vi "daq_sound_output.vi"() -> ()   [LabVIEW 2022 SP3]
uses:
  typedefs/state_control.ctl
  <vilib>/DAQmx/write.llb/DAQmx Write (Analog Wfm 1Chan NSamp).vi
  <vilib>/DAQmx/create/channels.llb/DAQmx Create Channel (AO-Voltage-Basic).vi
  <vilib>/sound2/lvsound2.llb/Sound File Read Open.vi
  <vilib>/sound2/lvsound2.llb/Sound File Info (refnum).vi
  <vilib>/DAQmx/configure/timing.llb/DAQmx Timing (Sample Clock).vi
  <vilib>/DAQmx/miscellaneous.llb/DAQmx Fill In Error Info.vi
panel:
  in  "Strain Gauge":tag="cDAQ4Mod1/ai0"
  in  "Thermocouple":tag="cDAQ4Mod2/ai0"
  in  "Play\nButton":bool
  in  "Trigger source in":tag="/cDAQ4/PFI0"
  in  "Trigger counter":tag="cDAQ4/_ctr0"
  in  "LEDs":tag="cDAQ4Mod3/port0/line0:7"
  in  "stop":bool
  in  "Path":path=path "C:/Users/Dell NI/Desktop/SoundEditor/data/39;SING, SING, SING39; BY BENNY GOODMAN-YoutubeConvert.cc.wav"
  in  "Audio Output":tag="cDAQ4Mod4/ao0"
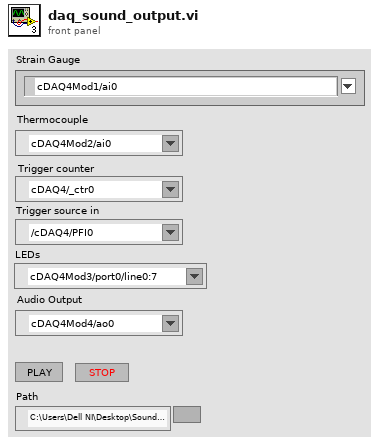
[diagram p1: front panel]
types:
  T1 = typedef "state_control.ctl" = enum16{"Running", "Stopped", "Forwarding"}
  T2 = typedef "Sound File Refnum.ctl" = refnum<file>
  T3 = typedef "Sound Data Format.ctl" = cluster{"sample rate (S/s)":dbl, "number of channels":i32, "bits per sample":i32}
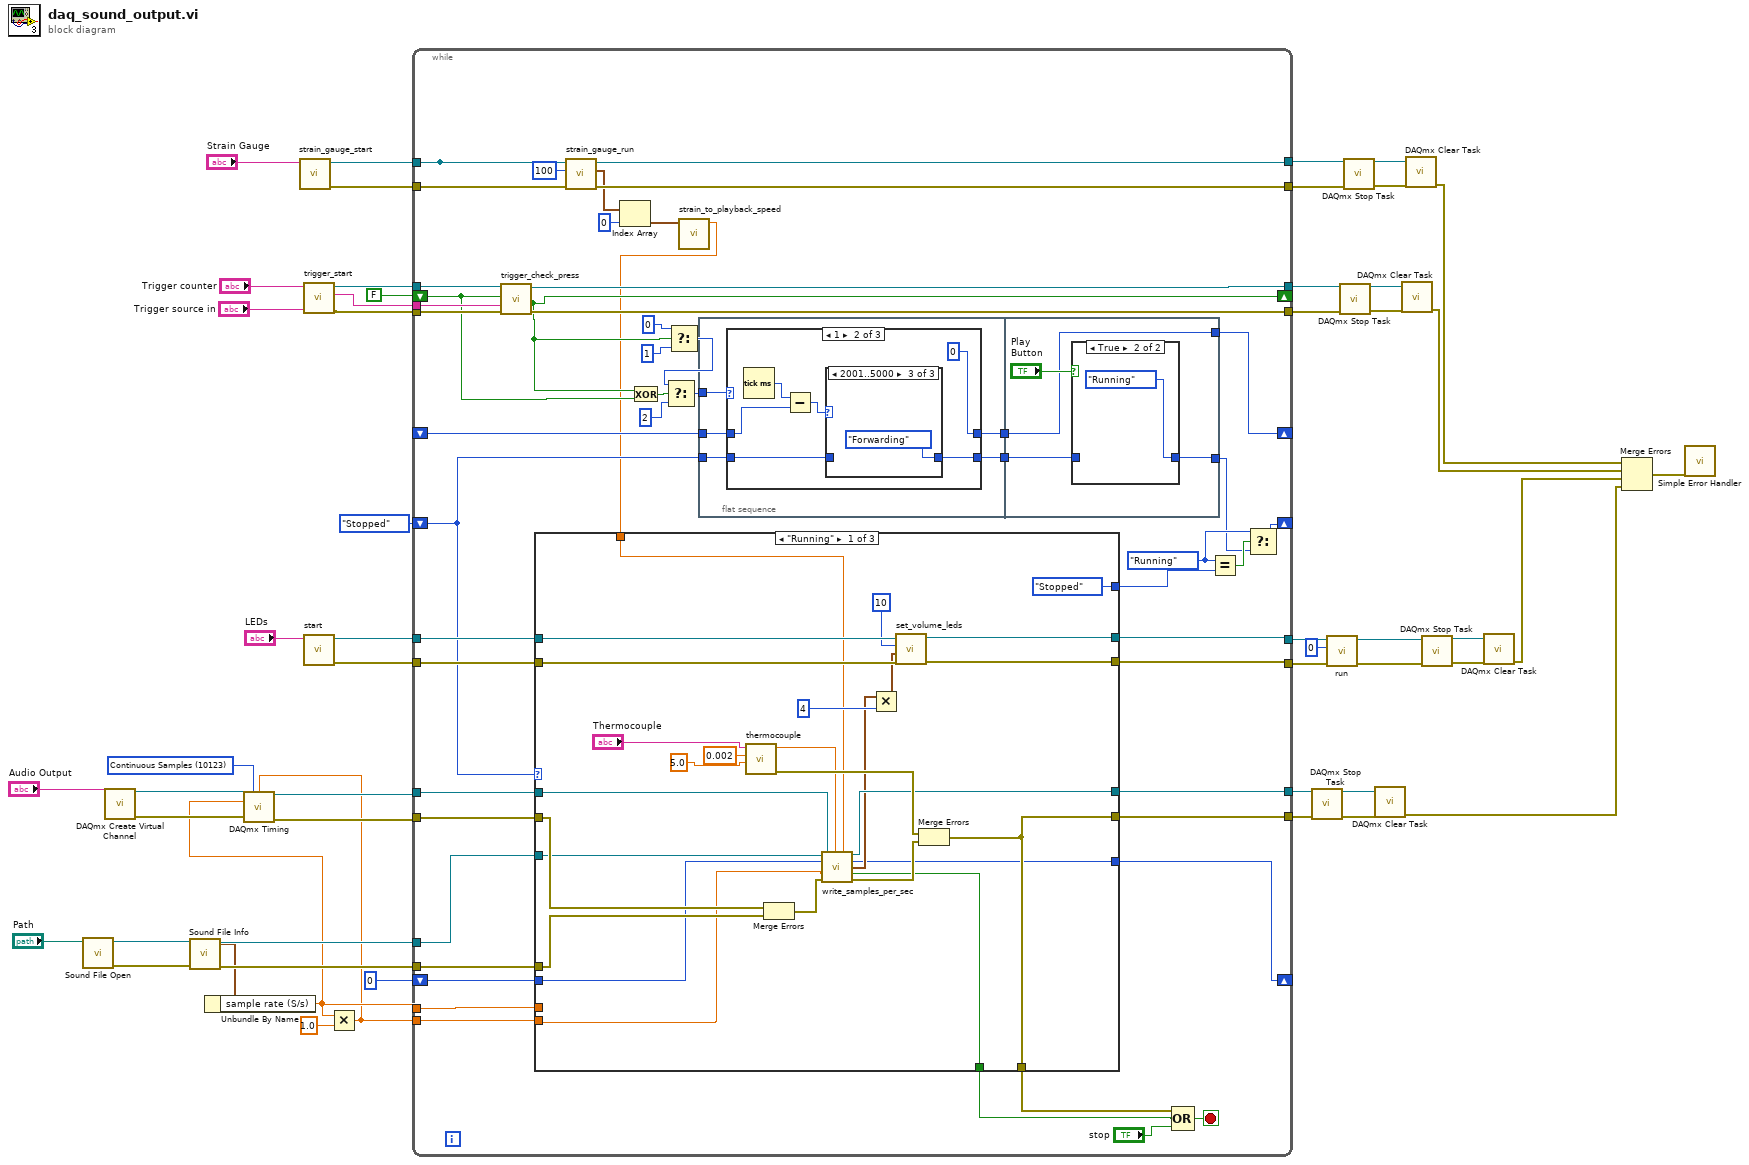
[diagram p0: block diagram]
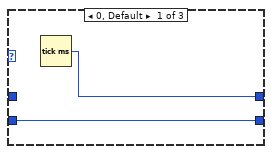
[diagram p2: hidden frame]
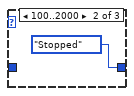
[diagram p4: hidden frame]
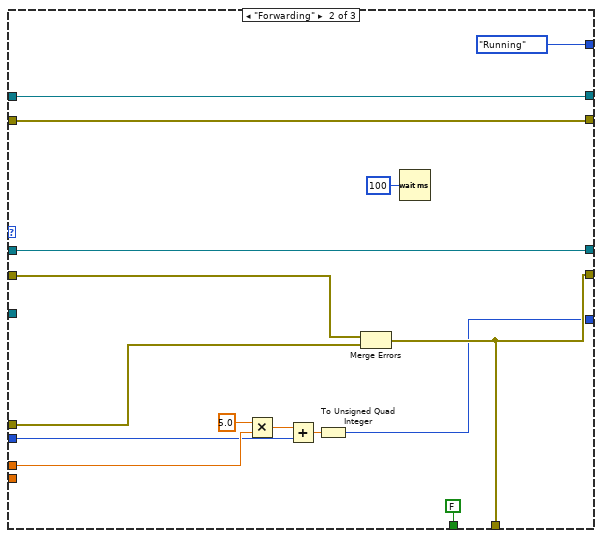
[diagram p7: hidden frame]
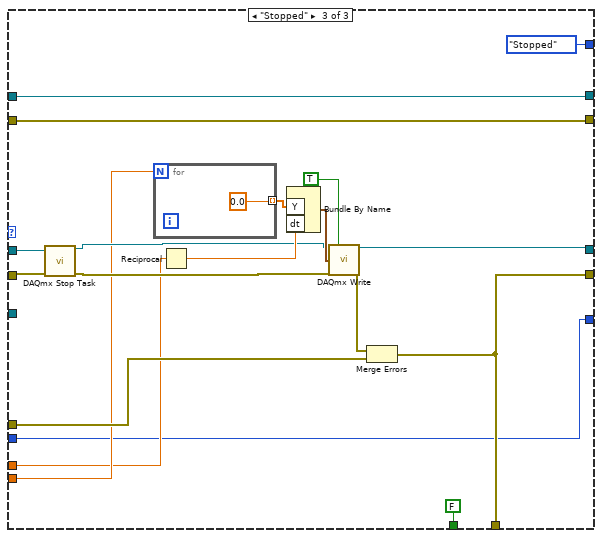
[diagram p8: hidden frame]
diagram:
  w38 = 10123 items=["Finite Samples"=10178, "Continuous Samples"=10123, "Hardware Timed Single Point"=12522] ("sample mode")
  n1 = call-poly <vilib>:"Sound File Open.vi"("path"="Path") -> ("error out"=w48:errorcluster, "sound file refnum"=w49:T2)  [unwired: 9 in]
  n2 = call-poly <vilib>:"DAQmx Create Virtual Channel.vi"("physical channels"="Audio Output") -> ("task out"=w44:refnum<k21>, "error out"=w43:errorcluster)  [unwired: 13 in]
  n3 = call-poly <vilib>:"Sound File Info.vi"("error in (no error)"=w48, "sound file refnum"=w49) -> ("error out"=w47:errorcluster, "sound format"=w45:T3, "sound file refnum out"=w46:T2)  [unwired: 6 in, 1 out]
  n4 = Unbundle By Name(w45) -> ("sample rate (S/s)"=w16:dbl)
  n5 = call "strain_gauge_start.vi"("Physical Channel"="Strain Gauge") -> ("error out"=w10:errorcluster, "task out"=w11:refnum<k21>)  [unwired: 8 in, 1 out]
  n6 = call "trigger_start.vi"("Trigger source in"="Trigger source in", "Trigger counter"="Trigger counter") -> ("error out"=w21:errorcluster, "Trigger source out"=w18:tag, "Refnum out"=w23:refnum<k21>)  [unwired: 7 in]
  n7 = call "start.vi"("lines"="LEDs") -> ("error out"=w34:errorcluster, "Refnum out"=w35:refnum<k21>)  [unwired: 9 in]
  n8 = Multiply(x=w16, y=1.0) -> (x*y=w15:dbl)
  n9 = call-poly <vilib>:"DAQmx Timing.vi"("task/channels in"=w44, "sample mode"=w38, "samples per channel"=w15, "rate"=w16, "error in"=w43) -> ("task out"=w42:refnum<k21>, "error out"=w41:errorcluster)  [unwired: 9 in]
  n10 = while {
    tunnel: w46 -> [w103]
    tunnel: w47 -> [w102]
    tunnel: w42 -> [w101]
    tunnel: w41 -> [w100]
    tunnel: w16 -> [w93]
    tunnel: [w98] -> w40
    tunnel: [w99] -> w39
    tunnel: w35 -> [w94]
    tunnel: w34 -> [w95]
    tunnel: [w97] -> w29
    tunnel: [w96] -> w28
    tunnel: w23 -> [w91]
    tunnel: [w89] -> w22
    tunnel: w21 -> [w92]
    tunnel: [w90] -> w20
    shift-right: [w85] -> _
    shift-left: FALSE -> [w81]
    tunnel: w18 -> [w88]
    shift-right: [w70] -> _
    shift-left: state_control."Stopped" -> [w76]
    shift-right: [w79] -> _
    shift-left: _ -> [w78]
    tunnel: w15 -> [w69]
    shift-right: [w63] -> _
    shift-left: 0 -> [w64]
    tunnel: [w61] -> _
    tunnel: w11 -> [w61]
    tunnel: w10 -> [w62]
    tunnel: [w59] -> w7
    tunnel: [w58] -> w6
    stop <- w65 stop-if-true
    w72 = enum16{"Running", "Stopped"}."Running" ("x")
    n11 = call "trigger_check_press.vi"("error in (no error)"=w92, "source"=w88, "was_pressed?"=w81, "Refnum in"=w91) -> ("error out"=w90:errorcluster, "is pressed?"=w85:bool, "Refnum out"=w89:refnum<k21>)  [unwired: 5 in]
    n12 = call "strain_gauge_run.vi"("error in"=w62, "Samples per Loop"=100, "task/channels in"=w61) -> ("error out"=w58:errorcluster, "Waveform Chart"=w57:waveform(dbl)[], "task out"=w59:refnum<k21>)  [unwired: 6 in]
    n13 = Index Array(array=w57, index=0) -> (element=w55:waveform(dbl))
    n14 = Exclusive Or(1:w81, 2:w85) -> (0:w86:bool)
    n15 = Select(t=u8 0, s=w85, f=u8 1 ("t")) -> (s? t:f=w82:u8)
    n16 = Select(t=w82, s=w86, f=u8 2 ("t")) -> (s? t:f=w80:u8)
    n17 = call "strain_to_playback_speed.vi"("Waveform"=w55) -> ("playback speed"=w54:dbl)  [unwired: 10 in]
    n18 = case shown="\"Running\"" w76 {
      tunnel: w103 -> [w137 _ _]
      tunnel: w102 -> [w140 w163 w186]
      tunnel: [w143 w161 w185] -> w68
      tunnel: w101 -> [w141 w169 w179]
      tunnel: w100 -> [w139 w162 w178]
      tunnel: [w143 w161 w185] -> w99
      tunnel: [w134 w169 w180] -> w98
      tunnel: [w154 w167 w188] -> w97
      tunnel: [w153 w168 w187] -> w96
      tunnel: w95 -> [w152 w168 w187]
      tunnel: w94 -> [w151 w167 w188]
      tunnel: w93 -> [_ w165 w172]
      tunnel: [enum16{"Running", "Stopped"}."Stopped" enum16{"Running", "Stopped"}."Running" enum16{"Running", "Stopped"}."Stopped"] -> w74
      tunnel: w69 -> [w136 _ w173]
      tunnel: [w133 FALSE ("end of file?") FALSE ("end of file?")] -> w66
      tunnel: w64 -> [w131 w157 w170]
      tunnel: [w130 w155 w170] -> w63
      tunnel: w54 -> [w128 _ _]
      frame "Running" {
        n19 = call "thermocouple.vi"("max volume"=5.0, "volume rise per 1C"=0.002, "physical channels"="Thermocouple") -> ("error out"=w144:errorcluster, "volume"=w142:dbl)  [unwired: 7 in]
        n20 = Merge Errors(w139, w140) -> (w138:errorcluster)
        n21 = call "write_samples_per_sec.vi"("Byte Stream File in"=w137, "task in"=w141, "Volume"=w142, "Playback speed"=w128, "Sample offset"=w131, "Samples per channel"=w136, "error in"=w138) -> ("Refnum out"=w134:refnum<k21>, "next_offset"=w130:u64, "data out"=w132:waveform(dbl), "end of file?"=w133:bool, "error out"=w135:errorcluster)  [unwired: 4 in]
        n22 = Multiply(x=w132, y=4) -> (x*y=w129:waveform(dbl))
        n23 = call "set_volume_leds.vi"("error in (no error)"=w152, "Array"=w129, "Numeric"=10, "Refnum in"=w151) -> ("error out"=w153:errorcluster, "Refnum out"=w154:refnum<k21>)  [unwired: 6 in]
        n24 = Merge Errors(w144, w135) -> (w143:errorcluster)
      }
      frame "Forwarding" {
        n25 = Multiply(x=5.0, y=w165) -> (x*y=w164:dbl)
        n26 = Add(x=w164, y=w157) -> (x+y=w156:dbl)
        n27 = To Unsigned Quad Integer(1:w156) -> (0:w155:u64)
        n28 = Merge Errors(w162, w163) -> (w161:errorcluster)
        n29 = Wait (ms)(milliseconds to wait=u32 100) -> ()  [unwired: 1 out]
      }
      frame "Stopped" {
        n30 = call <vilib>:"DAQmx Stop Task.vi"("task/channels in"=w179, "error in"=w178) -> ("task out"=w176:refnum<k21>, "error out"=w177:errorcluster)  [unwired: 12 in]
        n31 = for {
          N: w173 -> [_]
          tunnel: [0.0] -> w183 mode=indexing
        }
        n32 = Reciprocal(x=w172) -> (1/x=w184:dbl)
        n33 = Bundle By Name("Y"=w183, "dt"=w184) -> (w182:waveform(dbl))  [unwired: 1 in]
        n34 = call-poly <vilib>:"DAQmx Write.vi"("task/channels in"=w176, "auto start"=TRUE, "data"=w182, "error in"=w177) -> ("task out"=w180:refnum<k21>, "error out"=w181:errorcluster)  [unwired: 9 in, 1 out]
        n35 = Merge Errors(w181, w186) -> (w185:errorcluster)
      }
    }
    n36 = flat-sequence {
      tunnel: w80 -> [w108]
      tunnel: w78 -> [w106]
      tunnel: [w107] -> w77
      tunnel: w76 -> [w105]
      tunnel: [w104] -> w75
      tunnel: [w124] -> w79
      tunnel: w77 -> [w124]
      tunnel: [w122] -> w71
      tunnel: w75 -> [w123]
      frame #0 {
        n37 = case shown="1" w108 {
          tunnel: [w110 u32 0 ("millisecond timer value") w121] -> w107
          tunnel: w106 -> [_ w115 w121]
          tunnel: w105 -> [w109 w114 w120]
          tunnel: [w109 w112 w120] -> w104
          frame 0, Default {
            n38 = Tick Count (ms)() -> (millisecond timer value=w110:u32)
          }
          frame 1 {
            n39 = Tick Count (ms)() -> (millisecond timer value=w116:u32)
            n40 = Subtract(x=w116, y=w115) -> (x-y=w111:u32)
            n41 = case shown="2001..5000" w111 {
              tunnel: w114 -> [w117 _ _]
              tunnel: [w117 enum16{"Running", "Stopped"}."Stopped" state_control."Forwarding"] -> w112
              frame 0..99, Default {
              }
              frame 100..2000 {
              }
              frame 2001..5000 {
              }
            }
          }
          frame 2 {
          }
        }
      }
      frame #1 {
        n42 = case shown="True" "Play\nButton" {
          tunnel: [w126 enum16{"Running", "Stopped"}."Running"] -> w122
          tunnel: w123 -> [w126 _]
          frame False {
          }
          frame True {
          }
        }
      }
    }
    n43 = Compound Arithmetic op=OR(w68, w66, "stop") -> (w65:bool)
    n44 = Equal?(x=w72, y=w74) -> (x = y?=w73:bool)
    n45 = Select(t=w72, s=w73, f=w71) -> (s? t:f=w70:T1)
  }
  n46 = call <vilib>:"DAQmx Stop Task.vi"("task/channels in"=w40, "error in"=w39) -> ("task out"=w53:refnum<k21>, "error out"=w52:errorcluster)  [unwired: 12 in]
  n47 = call "run.vi"("error in (no error)"=w28, "volume"=0, "Refnum in"=w29) -> ("error out"=w31:errorcluster, "Refnum out"=w32:refnum<k21>)  [unwired: 7 in]
  n48 = call <vilib>:"DAQmx Stop Task.vi"("task/channels in"=w22, "error in"=w20) -> ("task out"=w25:refnum<k21>, "error out"=w24:errorcluster)  [unwired: 12 in]
  n49 = call <vilib>:"DAQmx Stop Task.vi"("task/channels in"=w7, "error in"=w6) -> ("task out"=w9:refnum<k21>, "error out"=w8:errorcluster)  [unwired: 12 in]
  n50 = call <vilib>:"DAQmx Clear Task.vi"("task in"=w53, "error in"=w52) -> ("error out"=w2:errorcluster)  [unwired: 13 in]
  n51 = call <vilib>:"DAQmx Clear Task.vi"("task in"=w25, "error in"=w24) -> ("error out"=w4:errorcluster)  [unwired: 13 in]
  n52 = call <vilib>:"DAQmx Clear Task.vi"("task in"=w9, "error in"=w8) -> ("error out"=w5:errorcluster)  [unwired: 13 in]
  n53 = call <vilib>:"DAQmx Stop Task.vi"("task/channels in"=w32, "error in"=w31) -> ("task out"=w37:refnum<k21>, "error out"=w36:errorcluster)  [unwired: 12 in]
  n54 = call <vilib>:"DAQmx Clear Task.vi"("task in"=w37, "error in"=w36) -> ("error out"=w3:errorcluster)  [unwired: 13 in]
  n55 = Merge Errors(w5, w4, w3, w2) -> (w1:errorcluster)
  n56 = call <vilib>:"Simple Error Handler.vi"("error in (no error)"=w1) -> ()  [unwired: 4 in, 5 out]
